vi "threshold.vi"   [LabVIEW 2015, in "binary_search.lvlib"]
uses:
  binary_search.lvlib
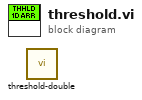
[diagram p0: block diagram]
diagram:
  n1 = call "threshold-double.vi"() -> ()  [unwired: 11 in, 1 out]
